vi "Microscope.GetDependencies.vi"(8 "error in (no error)":errorcluster, 11 "Microscope":refnum<class "Microscope.lvclass">) -> (0 "error out":errorcluster, 2 "Dependencies":T1, 3 "Microscope out":refnum<class "Microscope.lvclass">)   [LabVIEW 2013, in "Microscope.lvclass"]
doc: "---------------------------------------------------------------\nJKI State Machine Objects™\nhttp://jki.net/state-machine-objects/\nCopyright (C) 2005-2015, JKI <info@jki.net>\nALL RIGHTS RESERVEDJKI State Machine Objects (SMO) 1.0.0.5\nJKI - JKI\nCopyright (c) 2016, JKI"
uses:
  Microscope.lvclass
  Typedefs/Dependencies--Cluster.ctl
  XYStage/XYStage.lvclass
  Camera/Camera.lvclass
  <vilib>/JKI/JKI SMO/SMO/SMO.lvclass
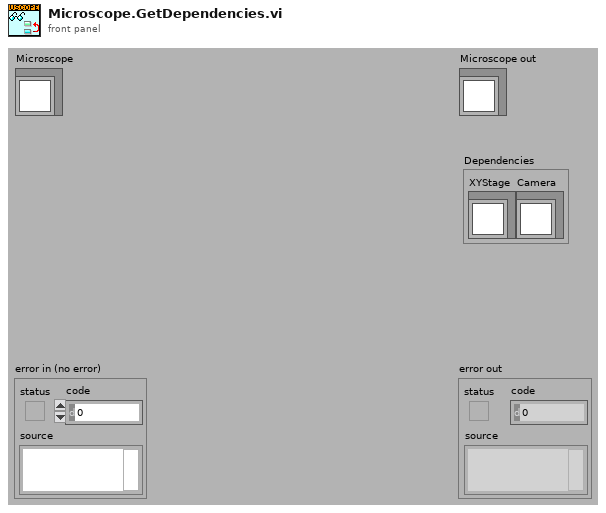
[diagram p1: front panel]
types:
  T1 = typedef "Microscope.lvclass/Dependencies--Cluster.ctl" = cluster{"XYStage":refnum<class "XYStage.lvclass">, "Camera":refnum<class "Camera.lvclass">}
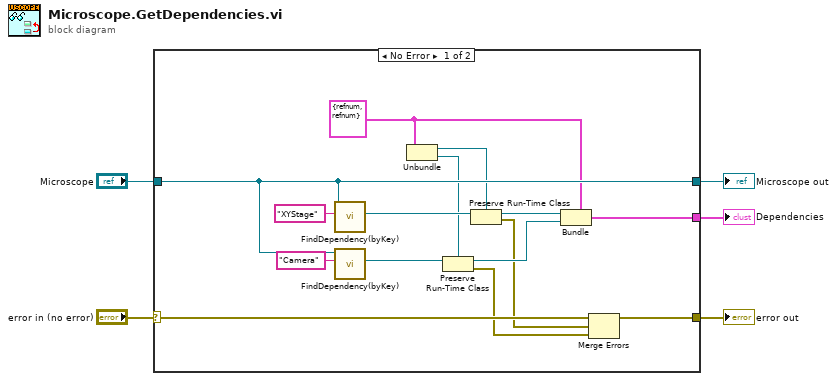
[diagram p0: block diagram]
diagram:
  n1 = case shown="No Error" "error in (no error)" {
    selector: "error in (no error)" -> [w19 w21]
    tunnel: "Microscope" -> [w17 w22]
    tunnel: [w18 w21] -> w5
    tunnel: [w17 w22] -> w4
    tunnel: [w20 _] -> w3
    frame No Error {
      w8 = T1 {"XYStage"=refnum, "Camera"=refnum} ("Dependencies")
      n2 = call <vilib>:"FindDependency(byKey).vi"("Key"="XYStage", "SMO in"=w17) -> ("Dependency"=w14:refnum<class "SMO.lvclass">)  [unwired: 6 in, 3 out]
      n3 = call <vilib>:"FindDependency(byKey).vi"("Key"="Camera", "SMO in"=w17) -> ("Dependency"=w11:refnum<class "SMO.lvclass">)  [unwired: 6 in, 3 out]
      n4 = Unbundle(w8) -> ("XYStage"=w12:refnum<class "XYStage.lvclass">, "Camera"=w10:refnum<class "Camera.lvclass">)
      n5 = Preserve Run-Time Class(object in=w11, 2:w10) -> (object out=w9:refnum<class "Camera.lvclass">, error out=w6:errorcluster)  [unwired: 1 in]
      n6 = Preserve Run-Time Class(object in=w14, 2:w12) -> (object out=w13:refnum<class "XYStage.lvclass">, error out=w7:errorcluster)  [unwired: 1 in]
      n7 = Bundle(cluster=w8, "XYStage"=w13, "Camera"=w9) -> (w20:T1)
      n8 = Merge Errors(w19, w7, w6) -> (w18:errorcluster)
    }
    frame Error {
      # "Upstream error or State Machine Object has not been created."
    }
  }
  "error out" <- w5
  "Microscope out" <- w4
  "Dependencies" <- w3
